vi "setV.vi"(0 "comp":dbl, 2 "voltage":dbl, 3 "SMU":dbl, 4 "VISA resource name":refnum<visa-resource-name>="GPIB0::16::INSTR") -> (1 "VISA resource name dup":refnum<visa-resource-name>)   [LabVIEW 2023]
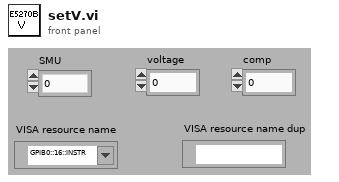
[diagram p1: front panel]
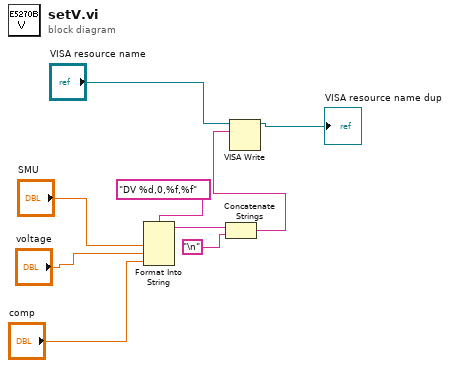
[diagram p0: block diagram]
diagram:
  n1 = Format Into String(format string="DV %d,0,%f,%f", "SMU", "voltage", "comp") -> (resulting string=w6:string)  [unwired: 2 in, 1 out]
  n2 = Concatenate Strings(w6, "\n") -> (w8:string)
  n3 = VISA Write(VISA resource name="VISA resource name", write buffer=w8) -> (VISA resource name out=→"VISA resource name dup":refnum<visa-resource-name>)  [unwired: 1 in, 2 out]
